vi "Apply Firmware.vi"(7 "System Credentials":T1, 8 "error in":errorcluster caption="error in (no error)", 11 "Target settings":T2={"Hostname"="", "Serial number"="", "Product name"="", "Product code"=0, "System status"="", "Credential type"=enum."None/Unlocked", "User added?"=FALSE, "Primary NIC"={"MAC address"="", "IP Address Request Mode"=2, "IP address"="", "Subnet mask"="", "Gateway"="", "DNS server"=""}} {"Primary NIC"."IP Address Request Mode" items=["Static"=1, "DHCP/Link-Local"=2, "Link-Local Only"=4, "DHCP Only"=8]}) -> (0 "error out":errorcluster, 2 "Detailed Result":string, 3 "Firmware Status":T4=2 items=["update pending auto restart"=-4, "verifying new image"=-3, "writing/flashing new image"=-2, "waiting for image"=-1, "corrupt firmware, cannot run"=0, "no firmware installed"=1, ""=2, "update pending user restart"=3, "update pending user action"=4, "update attempt failed"=5])   [LabVIEW 2020]
doc: "This Vi will upgrade the RT device's firmware if it is not supported by SystemLink Client, which means firmware must be higher than version 6."
uses:
  <vilib>/nisyscfg/Firmware Status.ctl
  SubVIs/Target Information.ctl
  subVIs/Targets/TypeDefs/rad_Target Network Settings.ctl
  SubVIs/System Credentials.ctl
  <vilib>/nisyscfg/Upgrade Firmware (File).vi
  <vilib>/nisyscfg/Close (Hardware).vi
  <vilib>/nisyscfg/Close (System).vi
  <resource>/objmgr/nisysapi.rc
  <vilib>/nisyscfg/nisyscfg.lvlib
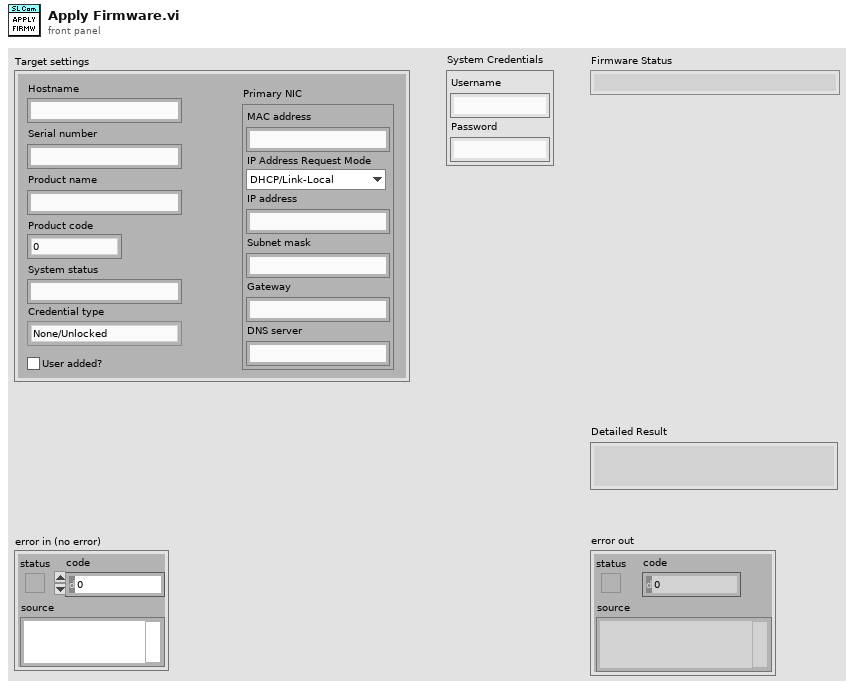
[diagram p1: front panel]
types:
  T1 = typedef "System Credentials.ctl" = cluster{"Username":string, "Password":string}
  T2 = typedef "Target Information.ctl" = cluster{"Hostname":string, "Serial number":string, "Product name":string, "Product code":i32, "System status":string, "Credential type":enum16{"None/Unlocked", "FTP Password", "NIAuth Credentials"}, "User added?":bool, "Primary NIC":T3}
  T3 = typedef "rad_Target Network Settings.ctl" = cluster{"MAC address":string, "IP Address Request Mode":i32, "IP address":string, "Subnet mask":string, "Gateway":string, "DNS server":string}
  T4 = typedef "nisyscfg.lvlib/Firmware Status.ctl" = i32
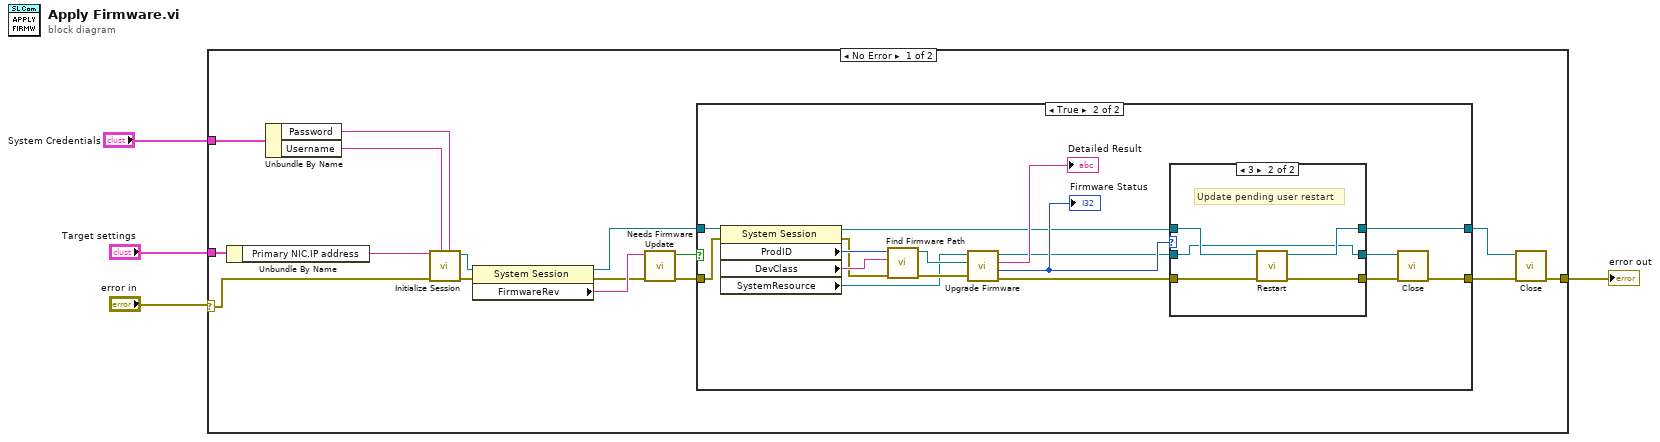
[diagram p0: block diagram]
diagram:
  n1 = case shown="No Error" "error in" {
    selector: "error in" -> [w11 w48]
    tunnel: [w20 w48] -> w2
    tunnel: "Target settings" -> [w17 _]
    tunnel: "System Credentials" -> [w7 _]
    frame No Error {
      n2 = Unbundle By Name(w17) -> ("Primary NIC.IP address"=w16:string)
      n3 = Unbundle By Name(w7) -> ("Password"=w5:string, "Username"=w6:string)
      n4 = call <vilib>:"Initialize Session.vi"("Password"=w5, "User Name"=w6, "error in (no error)"=w11, "Target (localhost)"=w16) -> ("error out"=w19:errorcluster, "Session out"=w18:refnum<k21>)  [unwired: 6 in]
      n5 = property class="System Session"(reference=w18, error in=w19) -> (reference out=w13:refnum<k21>, error out=w14:errorcluster, "FirmwareRev"=w15:string)
      n6 = call "Needs Firmware Update.vi"("error in (no error)"=w14, "FirmwareRev"=w15) -> ("error out"=w9:errorcluster, "Update?"=w10:bool)  [unwired: 8 in]
      n7 = case shown="True" w10 {
        tunnel: w9 -> [w21 w33]
        tunnel: w13 -> [w22 w34]
        tunnel: [w22 w36] -> w12
        tunnel: [w21 w25] -> w8
        frame False {
          # "RT device doesn't require a firmware update. It is already compatible with SystemLink Client."
        }
        frame True {
          n8 = property class="System Session"(reference=w34, error in=w33) -> (reference out=w27:refnum<k21>, error out=w30:errorcluster, "ProdID"=w32:i32, "DevClass"=w31:string, "SystemResource"=w23:refnum<k20>)
          n9 = call "Find Firmware Path.vi"("error in"=w30, "Device Class"=w31, "Product ID"=w32) -> ("error out"=w28:errorcluster, "Firmware Path"=w29:path)  [unwired: 7 in]
          n10 = call-poly <vilib>:"Upgrade Firmware.vi"("error in (no error)"=w28, "Firmware File"=w29, "Resource in"=w23) -> ("error out"=w38:errorcluster, "Firmware Status"=w37:T4, "Detailed Result"=→"Detailed Result":string, "Resource out"=w35:refnum<k20>)  [unwired: 5 in]
          "Firmware Status" <- w37
          n11 = case shown="3" w37 {
            tunnel: w38 -> [w41 w47]
            tunnel: w27 -> [w42 w46]
            tunnel: [w42 w45] -> w36
            tunnel: [w41 w44] -> w26
            tunnel: w35 -> [w40 w43]
            tunnel: [w40 w43] -> w24
            frame 0, Default {
            }
            frame 3 {
              # "Update pending user restart"
              n12 = call <vilib>:"Restart.vi"("error in (no error)"=w47, "Session in"=w46) -> ("error out"=w44:errorcluster, "Session out"=w45:refnum<k21>)  [unwired: 7 in, 1 out]
            }
          }
          n13 = call-poly <vilib>:"Close.vi"("error in (no error)"=w26, "Resource in"=w24) -> ("error out"=w25:errorcluster)  [unwired: 9 in]
        }
      }
      n14 = call-poly <vilib>:"Close.vi"("error in (no error)"=w8, "Session in"=w12) -> ("error out"=w20:errorcluster)  [unwired: 9 in]
    }
    frame Error {
    }
  }
  "error out" <- w2
